vi "Q_learning_Global.vi"() -> ()   [LabVIEW 2010]
panel:
  in  "step_counter":dbl
  in  "Parameter":T1={"N_STATES"=6.0, "EPSILON"=0.9, "ALPHA"=0.1, "GAMMA"=0.9, "MAX_EPISODES"=13.0, "FRESH_TIME"=0.3, "ACTIONS"=["left", "right"]}
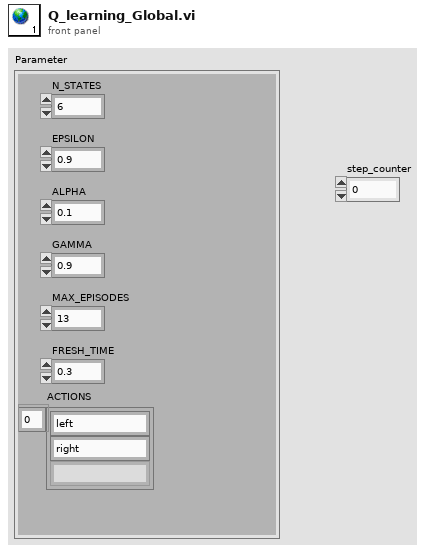
[diagram p1: front panel]
types:
  T1 = cluster{"N_STATES":dbl, "EPSILON":dbl, "ALPHA":dbl, "GAMMA":dbl, "MAX_EPISODES":dbl, "FRESH_TIME":dbl, "ACTIONS":string[]}
diagram:
